vi "UHR-Fleezers Control (host) - 12.1_Jonathan.vi"() -> ()   [LabVIEW 2012] (continued)
  in  "Save Trap Pos. Data":bool=TRUE
  in  "Lower Ch. Cap.":bool
  in  "Top 3 Harvard Syringe Pump Serial Port":refnum<visa-resource-name>="Top3Harvard"
  out "Database link":path
  out "Save Data Period (s)":dbl=0.00375 caption="Period (s)" format="%#_6p"
  out "Save Data Rate (Hz)":dbl=266.6666666666667 caption="Rate (Hz)" format="%#_6p"
  in  "Save ave N":dbl=250.0 caption="Averaging Factor"
  in  "Save N Sets":bool
  in  "N sets to save":u32=200 caption="N Sets"
  out "Total Time (s) 2":dbl=60.0
  # "After"
  # "During"
  # "Trap On?"
  # "BD Flow ON?"
  # "Samp Flow ON?"
  # "Trap Trig. Fl.?"
  # "Zero It"
  # "Floor it\n(e.g., hp unwinding)"
  # "1"
  # "2"
  # "Fl. Down"
  # "Fl. Up"
  # "Bead sep"
  # "Trap Display:"
  # "APD Display:"
  # "DAQ"
  # "Trap Manipulation"
  # "Data Saving"
  # "Bead Calibration"
  # "Bottom Pump (#1)"
  # "Central Sample Channels"
  # "Top Pump (#3)"
  # "Rate param is ul/h\nVolume param is ul"
  # "Chemyx Pump 2"
  # "Units: \n1 = ml/m\n2 = ml/h\n3 = ul/m\n4 = ul/h"
  # "X"
  # "Y"
  # "Oscillate Set 1 freq. (debugging)"
  # "BD 1"
  # "BD 2"
  # "AOD Raster Scan"
  # "Approx. trap separations"
  # "X"
  # "Y"
  # "FPGA\nreading"
  # "DMA\ntransfer"
  # "APD Gates"
  # "APD 2"
  # "APD 1"
  # "X"
  # "2D"
  # "Y"
  # "1D"
  # "Green Laser Interlacing"
  # "Green FB Measurement"
  # "Digital Gate"
  # "Current Analog Control"
  # "Total AI Rates (NOT rates/trap)"
  # "(Samples/trap x Trap Sets)"
  # "(Samples/channel x\n8 if averaging (8 channels)\n4 if no averaging)"
  # "Trap 1"
  # "Trap 2"
  # "Flour./Trap 3"
  # "External Video Window"
  # "MCL Position Debugging"
  # "Temporary Control Storage\n(these used to be somewhere else, still want to keep them)"
  # "Y"
  # "X"
  # "Trap Position Difference Limits"
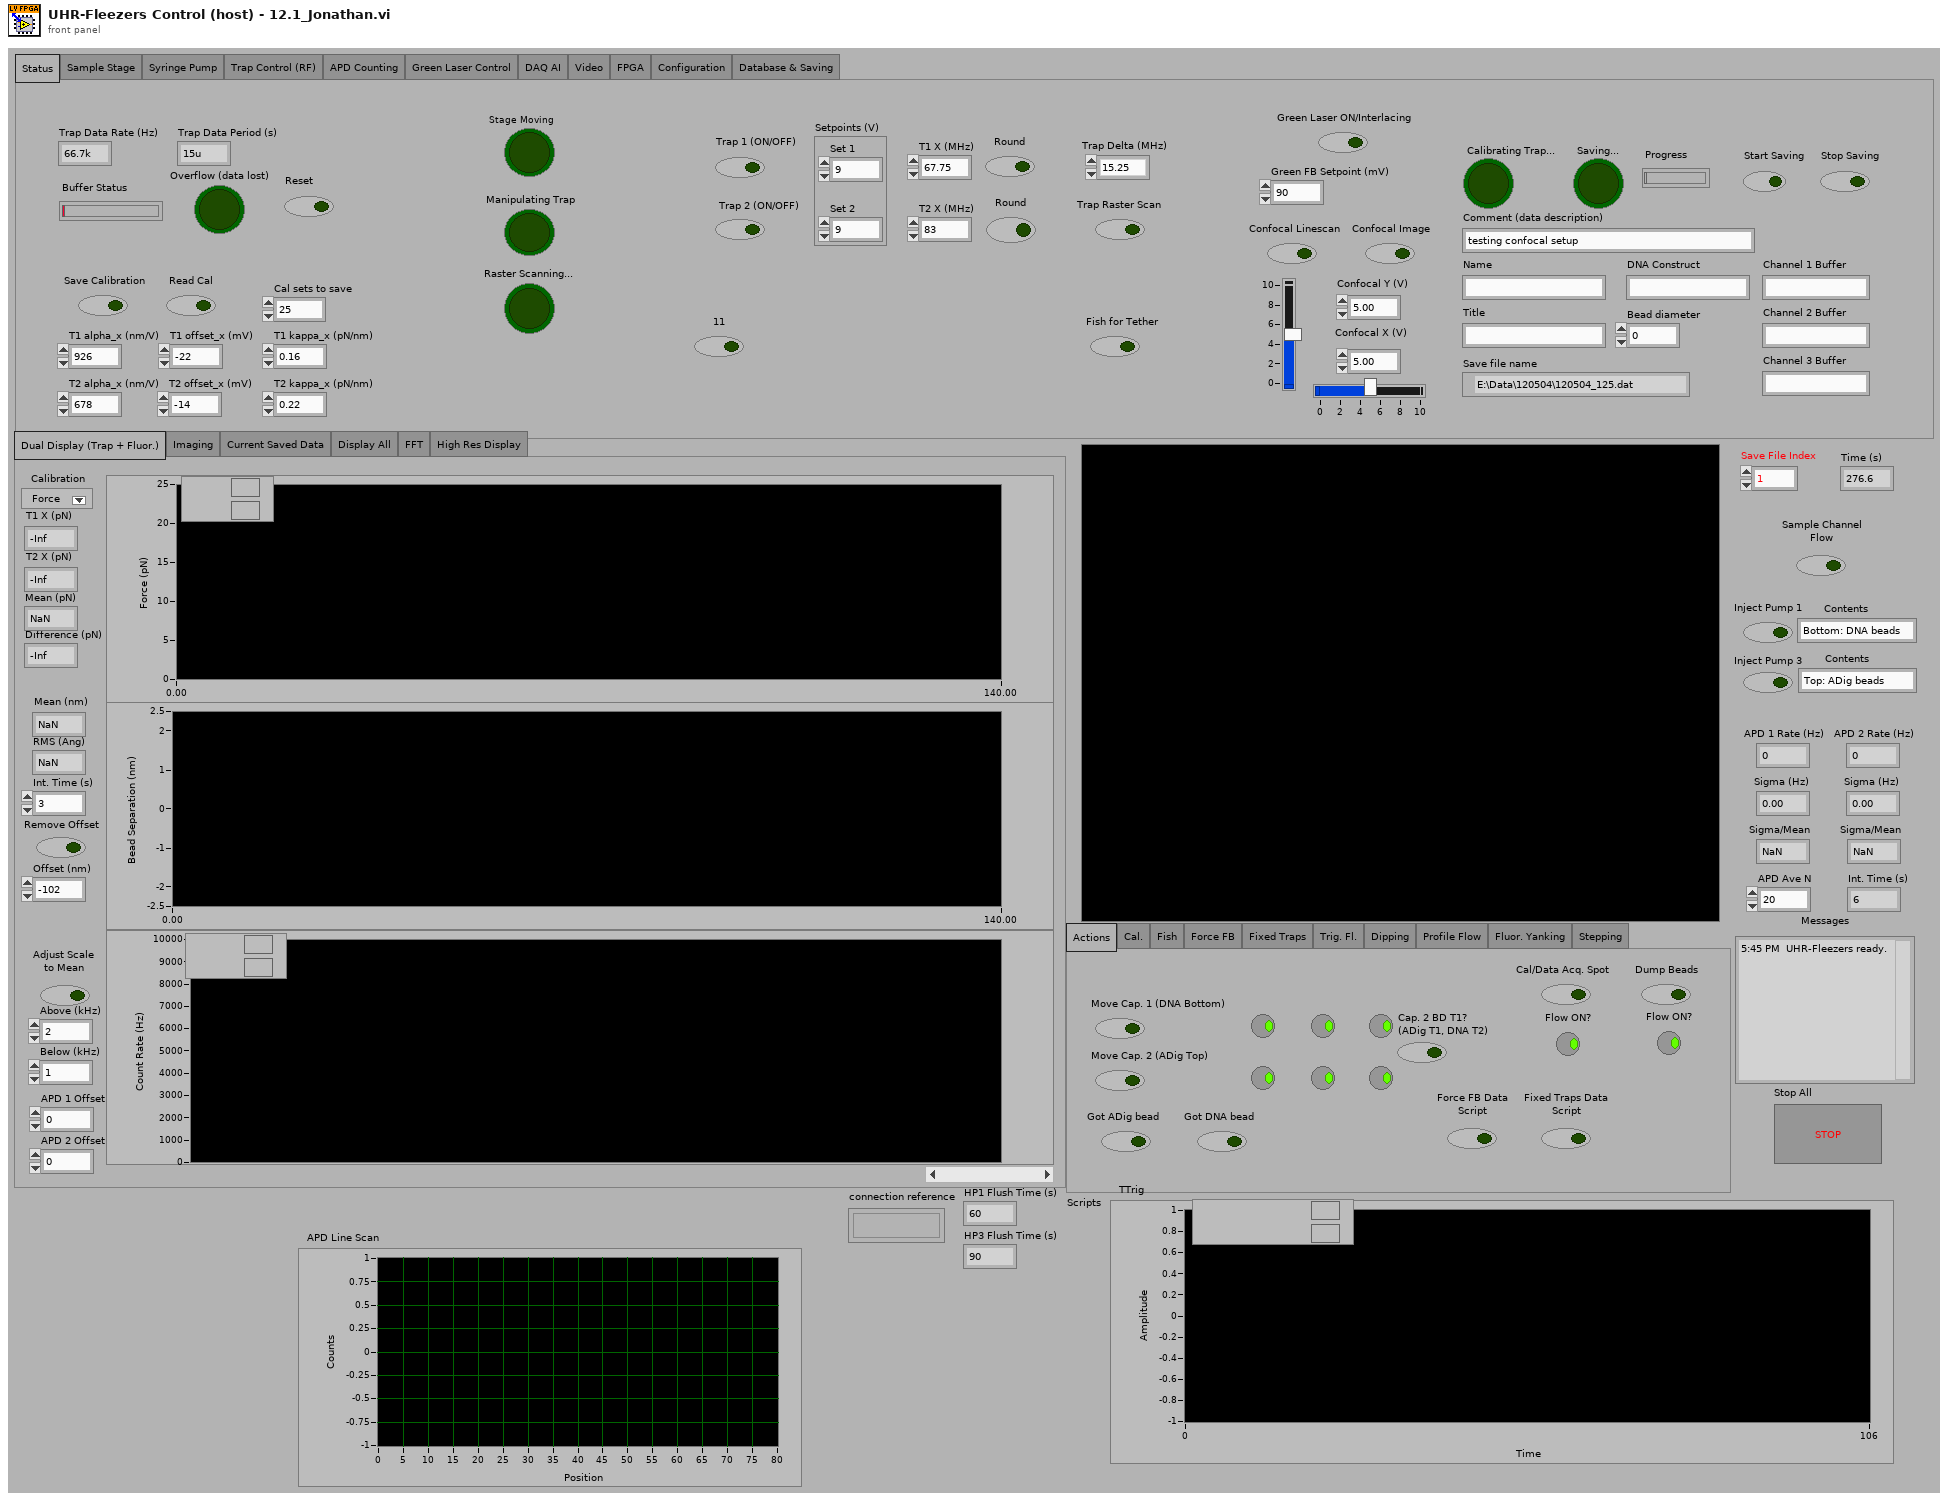
[diagram p1: front panel]
types:
  T1 = typedef "NI_Database_API.lvlib/Conn ObjectReference.ctl" = refnum<k1>
  T2 = enum32{"Actions", "Cal.", "Fish", "Force FB", "Fixed Traps", "Trig. Fl.", "Dipping", "Profile Flow", "Fluor. Yanking", "Stepping"}
  T3 = typedef "IMAQ Image.ctl" = refnum<image>
  T4 = enum32{"Dual Display (Trap + Fluor.)", "Imaging", "Current Saved Data", "Display All", "FFT", "High Res Display"}
  T5 = enum32{"Status", "Sample Stage", "Syringe Pump", "Trap Control (RF)", "APD Counting", "Green Laser Control", "DAQ AI", "Video", "FPGA", "Configuration", "Database & Saving"}
  T6 = cluster{"Pump 1":cluster{"Diameter (mm)":dbl, "Units":dbl, "Volume":dbl, "Rate":dbl}, "Pump 2":cluster{"Diameter (mm)":dbl, "Units":dbl, "Volume":dbl, "Rate":dbl}, "Pump 3":cluster{"Diameter (mm)":dbl, "Units":dbl, "Volume":dbl, "Rate":dbl}}
  T7 = enum32{"IR Laser Interlacing (Direct RF Board Control Method)", "AOD Raster Scan", "Feedback on Trap Intensity", "Feedback on Trap Position"}
  T8 = typedef "LVPoint32TypeDef.ctl" = cluster{"Horizontal":i32, "Vertical":i32}
  T9 = cluster{"Scan Range AOD (nm) 2":dbl, "Step Size AOD (nm) 2":dbl, "Scan Speed AOD (nm/s) 2":dbl, "Number of scans (AOD) 2":u16, "Label":string}[]
  T10 = cluster{"Set 1":cluster{"proportional gain (Kc)":i16, "integral gain (Kc*Ts/Ti)":i16, "derivative gain (Kc*Td/Ts)":i16}, "Set 2":cluster{"proportional gain (Kc)":i16, "integral gain (Kc*Ts/Ti)":i16, "derivative gain (Kc*Td/Ts)":i16}}
  T11 = cluster{"Trap 1":fxp<+/-,16,1>, "Trap 2":fxp<+/-,16,1>}
  T12 = cluster{"proportional gain (Kc)":fxp<+/-,16,8>, "integral gain (Kc*Ts/Ti)":fxp<+/-,16,8>, "derivative gain (Kc*Td/Ts)":fxp<+/-,16,8>}
  T13 = cluster{"output high":fxp<+/-,16,1>, "output low":fxp<+/-,16,1>}
  T14 = cluster{"Set 1":fxp<+/-,16,1>, "Set 2":fxp<+/-,16,1>}
  T15 = cluster{"proportional gain (Kc)":i16, "integral gain (Kc*Ts/Ti)":i16, "derivative gain (Kc*Td/Ts)":i16}
  T16 = cluster{"Set 1":bool, "Set 2":bool, "Set 3":bool}
  T17 = typedef "LVMinMaxIncTypeDef.ctl" = cluster{"Minimum":dbl, "Maximum":dbl, "Increment":dbl}
  T18 = typedef "Image Type" = u32
  T19 = typedef "nirio_resource_hc.ctl" = tag
  T20 = typedef "openfpgaref.8.6.ctl" = refnum<k20>
  T21 = cluster{"New Image":T3, "New Image":T3, "New Image":T3, "New Image":T3}
  T22 = typedef "XDNodeRunTimeDep.lvlib/timing_clust.ctl" = cluster{"Expected End [f-1]":u64, "Actual End [f-1]":u64, "Finished Late? [f-1]":bool, "Expected End [i-1]":u64, "Actual End [i-1]":u64, "Finished Late? [i-1]":bool, "Expected Start [i]":u64, "Actual Start [i]":u64, "Expected Start [f]":u64, "Actual Start [f]":u64, "Source Name":string, "Structure Name":string, "Period":i64, "Deadline":i64, "Offset":i64, "Start":i64, "Priority":i32, "Timeout":i32, "Mode":T23, "Wakeup Reason":T24, "Error":errorcluster, "Source Type":string, "Secondary Source Type":string, "Global End Time":u64, "Global Start Time":u64, "Frame Duration":u64, "Iteration Duration":u64, "Assigned CPU":i32, "I/O Scan Engine Mode":u32}
  T23 = typedef "XDNodeRunTimeDep.lvlib/nitl_modes.ctl" = enum32{"No Change", "Process missed periods, maintain original phase", "Discard missed periods, maintain original phase", "Process missed periods, ignore original phase", "Discard missed periods, ignore original phase"}
  T24 = typedef "XDNodeRunTimeDep.lvlib/wakeup.ctl" = enum32{"Normal", "Aborted", "Asynchronous wakeup", "Timing source error", "Timed loop error", "Timeout"}
  T25 = cluster{"Left":i32, "Top":i32, "Width":u32, "Height":u32}
  T26 = cluster{cluster{"Left":i32, "Top":i32, "Width":u32, "Height":u32}}[]
  T27 = enum32{"Status", "Sample Stage", "Syringe Pump", "Trap Control (RF)", "APD Counting", "Green Laser Control", "DAQ AI", "Video", "FPGA", "Configuration"}
  T28 = enum32{"setting", "request", "request control", "info", "statistics", "system settings", "I/O sub system", "HRT control", "camera descriptions", "device specific data", "event sub system settings", "event sub system results", "image memory manager"}
  T29 = typedef "AviRefnum.ctl" = refnum<k1>
  T30 = typedef "imagedata.ctl" = cluster{"image type":i32, "image depth":i32, "image":u8[], "mask":u8[], "colors":u32[], "Rectangle":cluster{"left":i16, "top":i16, "right":i16, "bottom":i16}}
  T31 = enum32{"Normal Display", "Dual Display (APD)", "FFT", "High Res Display"}
  T32 = cluster{"Origin Pixel":cluster{"X":sgl, "Y":sgl}, "Angle Relative to Horizontal (deg)":sgl, "Axis Reference":u32}
  T33 = typedef "Simple Grid Descriptor" = cluster{"X Step":sgl, "Y Step":sgl, "Unit":T34}
  T34 = typedef "Image Unit" = enum32{"Undefined", "Angström", "Micrometer", "Millimeter", "Centimeter", "Meter", "Kilometer", "Microinch", "Inch", "Feet", "Nautical miles", "Standard miles", "Steps"}
  T35 = cluster{"averaging mode":u16, "weighting mode":u16, "number of averages":u32}
  T36 = cluster{"dB On (F)":bool, "unwrap phase (F)":bool, "convert to degree (F)":bool}
  T37 = enum16{"open", "replace", "create", "open or create", "replace or create", "replace or create with confirmation"}
  T38 = enum16{"big-endian, network order", "native, host order", "little-endian"}
  T39 = cluster{string, string, string, string, string, string, string, string}
  T40 = cluster{string, string, string, string, string, string, string, string, string, string, string, string}
  T41 = cluster{string, string, string, string, string, string, string, string, string, string, string, string, string}
  T42 = cluster{string, string, string, string, string, string, string, string, string, string, string, string, string, string}
  T43 = cluster{"BD 1 Frequency 1 (MHz)":dbl, "BD 1 Frequency 2 (MHz)":dbl}
  T44 = cluster{"f0":dbl, "df":dbl, "magnitude":dbl[]}[][]
  T45 = cluster{"Green FB Ch 0":i16, "Green FB Ch 1":i16, "Green FB Ch 2":i16}
  T46 = cluster{"Green FB Ch 0":dbl, "Green FB Ch 1":dbl, "Green FB Ch 2":dbl}
  T47 = cluster{"Comment (data description)":string, "Channel 1 Buffer":string, "Channel 2 Buffer":string, "Channel 3 Buffer":string, "Title":string, "DNA Construct":string, "Bead diameter":dbl, "Name":string}
  T48 = cluster{"Scan Range AOD (nm) 2":dbl, "Step Size AOD (nm) 2":dbl, "Scan Speed AOD (nm/s) 2":dbl, "Number of scans (AOD) 2":u16, "Label":string}
  T49 = cluster{"[0]":dbl, "[1]":dbl, "[2]":dbl, "[3]":dbl, "[4]":dbl, "[5]":dbl}
  T50 = cluster{"Diameter (mm)":dbl, "Units":dbl, "Volume":dbl, "Rate":dbl}
diagram:
  w14 = u16 20 items=["1.0"=10, "1.5"=15, "2.0"=20] ("stop bits (10: 1 bit)")
  w17 = u16 20 items=["1.0"=10, "1.5"=15, "2.0"=20] ("stop bits (10: 1 bit)")
  w74 = u16 20 items=["1.0"=10, "1.5"=15, "2.0"=20] ("stop bits (10: 1 bit)")
  w81 = T18 2 items=["Grayscale (U8)", "Grayscale (I16)", "Grayscale (SGL)", "Complex (CSG)", "RGB (U32)", "HSL (U32)", "RGB (U64)", "Grayscale (U16)"] ("Image Type")
  w143 = cluster{"output high":i16, "output low":i16} {"output high"=3000, "output low"=0} ("FB output range 1")
  w214 = 10.0 ("y")
  w213 = 32767.0 ("y")
  w229 = 6.0  # clock mult.
  w230 = 49152000.0  # TCXO frequ.
  # "Bottom 1 Harvard"
  # "Top 3 Harvard"
  # "Center Harvard"
  # "Bottom 1 Harvard"
  # "Top 3 Harvard"
  # "Center Harvard"
  n1 = Build Array("DIO count 1 (ticks)", "DIO count 2 (ticks)", "DIO count 3 (ticks)") -> (w131:u32[])
  n2 = local read "AO1"() -> (w208:dbl)
  n3 = local read "AO2"() -> (w207:dbl)
  n4 = local read "Scan Increment (MHz)"() -> (w225:dbl)
  n5 = local read "Continuous MCL Scanning"() -> (w195:bool)
  n6 = local read "Fast Scan Dir"() -> (w194:bool)
  n7 = local read "Number of scans (MCL)"() -> (w196:u64)
  n8 = property on="AI Count (ticks)" class="DigNum (strict)"("Val(Sgnl)"="AI Count (ticks)") -> ()  [unwired: 2 in, 2 out]
  n9 = Multiply(x=w208, y=w213) -> (x*y=w210:dbl)
  n10 = Multiply(x=w207, y=w213) -> (x*y=w212:dbl)
  n11 = Divide(x=w210, y=w214) -> (x/y=w209:dbl)
  n12 = Divide(x=w212, y=w214) -> (x/y=w211:dbl)
  n13 = To Word Integer(number=w209) -> (16bit integer=w206:i16)
  n14 = To Word Integer(number=w211) -> (16bit integer=w205:i16)
  n15 = Not(x=w194) -> (.not. x?=w189:bool)
  n16 = local read "Cycles/step (MCL)"() -> (w197:u64)
  n17 = Multiply(x=w225, y=1000.0) -> (x*y=w232:dbl)
  n18 = local read "Scan steps (MCL)"() -> (w198:u64)
  n19 = local write "Trap Pos FIFO Timeout"(u16 0 ("Trap Pos FIFO Timeout")) -> ()
  n20 = local read "Desired Scan Incr (V)"() -> (w200:dbl)
  n21 = Scale By Power Of 2(n=48, x=w232) -> (x*2^n=w233:dbl)
  n22 = Multiply(x=w230, y=w229) -> (x*y=w228:dbl)
  n23 = Divide(x=w233, y=w228) -> (x/y=w227:dbl)
  n24 = local read "Setpoints (V)"() -> (w246:cluster{"Set 1":dbl, "Set 2":dbl})
  n25 = To Quad Integer(1:w227) -> (0:w224:i64)
  n26 = Divide(x=40000000.0, y="AI Count (ticks)") -> (x/y=w185:dbl)
  n27 = Multiply(x=w200, y=32767.0) -> (x*y=w202:dbl)
  n28 = local read "Number Interlace Sets"() -> (w124:u8)
  n29 = Split 1D Array(array=w131, index=w124) -> (first subarray=w133:u32[])  [unwired: 1 out]
  n30 = Add Array Elements(numeric array=w133) -> (sum=w132:u32)
  n31 = local read "# Samples/channel"() -> (w217:u32)
  n32 = local read "Number of F/B Scans (AOD)"() -> (w218:u16)
  n33 = local read "Not-Interlacing Set"() -> (w123:enum32{"Set 1", "Set 2", "Set 3"})
  n34 = To Unsigned Byte Integer(number=w123) -> (unsigned 8bit integer=w129:u8)
  n35 = Index Array(array=w131, index=w129) -> (element=w130:u32)
  n36 = local read "Feedback On/Off"() -> (w249:cluster{"Set 1":bool, "Set 2":bool})
  n37 = local read "PID Gains"() -> (w241:T10)
  n38 = local read "Scan steps (AOD)"() -> (w223:u64)
  n39 = local read "All FB On/Off"() -> (w250:bool)
  n40 = local read "Cycles/step (AOD)"() -> (w222:u64)
  n41 = local write "AI rate (Hz)"(w185) -> ()
  n42 = Divide(x=w202, y=10.0) -> (x/y=w201:dbl)
  n43 = Multiply(x=w223, y=w222) -> (x*y=w221:u64)
  n44 = Multiply(x=3276.7, y=w246) -> (x*y=w245:cluster{"Set 1":dbl, "Set 2":dbl})
  n45 = xnode "FPGA Open VI Reference"("resource name"=T19 "750kHzDAQ") -> ("FPGA VI Reference Out"=w238:T20, "error out"=w237:errorcluster)  [unwired: 1 in]
  n46 = To Word Integer(number=w201) -> (16bit integer=w199:i16)
  n47 = Multiply(x=w221, y=u64 2) -> (x*y=w219:u64)
  n48 = local read "Sets to FIFO (Traps)"() -> (w253:T16)
  n49 = Divide(x=w185, y="FPGA Ave.") -> (x/y=w186:dbl)
  n50 = To Word Integer(number=w245) -> (16bit integer=w244:cluster{"Set 1":i16, "Set 2":i16})
  n51 = Unbundle By Name(w241) -> ("Set 1"=w240:T15, "Set 2"=w239:T15)
  n52 = Multiply(x=w219, y=w218) -> (x*y=w216:u64)
  n53 = local write "Ave. Rate (Hz)"(w186) -> ()
  n54 = Divide(x=w216, y=w217) -> (x/y=w215:dbl)
  n55 = Unbundle By Name(w244) -> ("Set 1"=w243:i16, "Set 2"=w242:i16)
  n56 = local read "2D or 1D Scan"() -> (w144:bool)
  n57 = local write "Data points/scans"(w216) -> ()
  n58 = local read "Scan BD"() -> (w234:bool)
  n59 = And(x=w249, y=w250) -> (x .and. y?=w248:cluster{"Set 1":bool, "Set 2":bool})
  n60 = local write "Data points/scan (f/b)"(w219) -> ()
  n61 = Reciprocal(x=w186) -> (1/x=w187:dbl)
  n62 = local read "N Acq Sets (Traps + Fl.)"() -> (w178:i16)
  n63 = local write "N sets should be saved"(w215) -> ()
  n64 = xnode "Invoke Method"("FPGA VI Reference In"=w238, "error in"=w237) -> ("FPGA VI Reference Out"=w142:T20, "error out"=w152:errorcluster)
  n65 = Unbundle By Name(w248) -> ("Set 1"=w252:bool, "Set 2"=w251:bool)
  n66 = local read "Interlace"() -> (w125:bool)
  n67 = Select(t=w132, s=w125, f=w130) -> (s? t:f=w122:u32)
  n68 = local write "Update Count (MCL)"(w122) -> ()
  n69 = local write "Total Counts (ticks)"(w122) -> ()
  n70 = local write "Ave. Period (s)"(w187) -> ()
  n71 = property on="2D or 1D Scan" class="Bool (strict)"("Val(Sgnl)"=w144) -> ()  [unwired: 2 in, 2 out]
  n72 = local read "GI Frequency, OFF count"() -> (w46:u32)
  n73 = local read "GI Frequency, ON count"() -> (w37:u32)
  n74 = local read "APD Gate OFF Count"() -> (w43:u32)
  n75 = local read "APD Gate ON Count"() -> (w39:u32)
  n76 = xnode "Read/Write Control"("FPGA VI Reference In"=w141, "error in"=w152, "ai count"="AI Count (ticks)", "Interlace ON/OFF"=w125, "Number Interlace Cycles"=w124, "AI1 Sets to FIFO"=w253, "FB On/Off Set 1"=w252, "FB On/Off Set 2"=w251, "Interlace Off Parameters"=w123, "FB Setpoint Set 1"=w243, "FB Setpoint Set 2"=w242, "FB Gains Set 1"=w240, "FB Gains Set 2"=w239, "FB output range 1"=w143, "FB output range 2"=w143, "Cycles per step"=w222, "Scan BD"=w234, "Number of scans"=w218, "Scan steps"=w223, "Scan freq.  increment"=w224, "AO1"=w206, "AO2"=w205, "Scan freq.  increment (MCL)"=w199, "Scan steps (MCL)"=w198, "Cycles per step (MCL)"=w197, "Number of scans (MCL)"=w196, "MCL count"=w122, "Cont. Scan (MCL)"=w195, "MCL Scan Axis"=w189, "1D or 2D Scan?"=w144, "N of AI1 Int Acq Sets"=w178, "Freq or Amp switch first"="Freq or Amp switch first", "Freq switch delay"="Freq switch delay", "Amp switch delay"="Amp switch delay", "Swap F1 and F2"="Swap F1 and F2", "APD to FIFO"=FALSE, "DIO count 1 (ticks)"="DIO count 1 (ticks)", "DIO count 2 (ticks)"="DIO count 2 (ticks)", "DIO count 3 (ticks)"="DIO count 3 (ticks)") -> ("FPGA VI Reference Out"=w50:T20, "error out"=w48:errorcluster)  [unwired: 1 in]
  n77 = local read "On one out of X cycles"() -> (w45:u32)
  n78 = local read "APD Integration Time (s)"() -> (w29:dbl)
  n79 = local read "DMA Update Period (s)"() -> (w28:dbl)
  n80 = Add(x=w39, y=w43) -> (x+y=w41:u32)
  n81 = Add(x=w37, y=w46) -> (x+y=w44:u32)
  n82 = local read "Green Laser ON/Interlacing"() -> (w120:bool)
  n83 = local read "Green laser mode"() -> (w121:enum32{"Laser ON", "Laser OFF", "Interlace"})
  n84 = Multiply(x=w41, y=w45) -> (x*y=w42:u32)
  n85 = Multiply(x=w45, y=w44) -> (x*y=w36:u32)
  n86 = Reciprocal(x=w29) -> (1/x=w26:dbl)
  n87 = Multiply(x=w29, y=40000000.0) -> (x*y=w25:dbl)
  n88 = Divide(x=w28, y=w29) -> (x/y=w31:dbl)
  n89 = Multiply(x="Current When FB OFF (%)", y=655.35) -> (x*y=w108:dbl)
  n90 = local read "Invert APD Gate"() -> (w35:bool)
  n91 = Multiply(x="Green FB Setpoint (mV)", y=3.2767) -> (x*y=w105:dbl)
  n92 = local read "APD Gate"() -> (w34:enum32{"ON", "OFF", "Interlace"})
  n93 = Subtract(x=w42, y=w39) -> (x-y=w40:u32)
  n94 = local write "Green FB Count"(w36) -> ()
  n95 = local write "APD Acq Rate (Hz)"(w26) -> ()
  n96 = To Unsigned Long Integer(number=w25) -> (unsigned 32bit integer=w23:u32)
  n97 = Multiply(x=2.0, y=w31) -> (x*y=w30:dbl)
  n98 = local read "Invert GI"() -> (w117:bool)
  n99 = To Unsigned Word Integer(number=w108) -> (unsigned 16bit integer=w106:u16)
  n100 = Subtract(x=w36, y=w37) -> (x-y=w38:u32)
  n101 = local write "APD Samples/FIFO Acq."(w31) -> ()
  n102 = To Word Integer(number=w105) -> (16bit integer=w103:i16)
  n103 = local write "APD Elements/DMA read"(w30) -> ()
  n104 = case shown="False" w120 {
    tunnel: w121 -> [_ w279]
    tunnel: [enum32{"Laser ON", "Laser OFF", "Interlace"}."Laser OFF" ("Green laser mode") w279] -> w116
    frame False {
    }
    frame True {
    }
  }
  n105 = local write "APD Int. Count"(w23) -> ()
  n106 = local read "Trap Pos. AI1 X Pre-scale"() -> (w60:u16)
  n107 = local read "Trap Pos FB Monitor\nT1 or T2"() -> (w67:bool)
  n108 = local read "Trap Pos FB Int Count"() -> (w54:u16)
  n109 = local read "APD 1 AO Mult."() -> (w33:i16)
  n110 = local read "Trap Pos FB Negate Action"() -> (w66:bool)
  n111 = local read "APD 2 AO Mult."() -> (w32:i16)
  n112 = local read "Trap Pos. FB Offset Factor"() -> (w65:i64)
  n113 = local read "Trap Pos. FB Mult Factor"() -> (w64:i64)
  n114 = local read "Differential FB?"() -> (w20:bool)
  n115 = local read "Neg. TTrig FPGA"() -> (w22:bool)
  n116 = local read "Trap Pos. FB Gains"() -> (w62:T12)
  n117 = local read "Trap Pos. FB Range"() -> (w63:T13)
  n118 = xnode "Read/Write Control"("FPGA VI Reference In"=w50, "error in"=w48, "Invert APD Gate"=w35, "APD Gate ON Count"=w39, "APD Gate OFF Count"=w40, "APD Acq Rate Count"=w23, "APD Gate Operating Mode"=w34, "APD 1 AO scale factor"=w33, "APD 2 AO scale factor"=w32, "Green interlace ON count"=w37, "Green interlace OFF count"=w38, "Green interlace ON count 2"=w37, "Green interlace OFF count 2"=w38, "Green FB Count"=w36) -> ("FPGA VI Reference Out"=w49:T20, "error out"=w47:errorcluster)
  n119 = xnode "Read/Write Control"("FPGA VI Reference In"=w49, "error in"=w47, "Invert GI 2"=w117, "Operating Mode 2"=w116, "Green FB Gains"="Green FB Gains", "Green FB Setpoint"=w103, "Green FB On/Off"="Green FB On/Off", "Current Out"=w106, "Green int current ON count adj"="Green int current ON count adj", "Operating Mode"=w116, "Invert GI"=w117, "Trap Pos FB Monitor T1 or T2"=w67, "Trap Pos FB Negate Action"=w66, "Trap Pos. FB Offset Factor"=w65, "Trap Pos. FB Mult Factor"=w64, "Trap Pos. FB Range"=w63, "Trap Pos. FB Gains"=w62, "Force feedback"=FALSE, "AI1 X Scale"=w60, "Trap Pos to FIFO"=TRUE, "Trap Pos FB Int Count"=w54, "TTrig Negate Pos"=w22, "FB Trig Integrate"="FB Trig Integrate", "Diff FB Measurement?"=w20, "Negate Diff?"="Negate Diff?") -> ("FPGA VI Reference Out"=w118:T20, "error out"=w119:errorcluster)
  n120 = xnode "Invoke Method"("FPGA VI Reference In"=w118, "error in"=w119, "Requested Depth"="Trap AI FIFO Depth") -> ("FPGA VI Reference Out"=w70:T20, "error out"=w69:errorcluster)  [unwired: 1 out]
  n121 = xnode "Invoke Method"("FPGA VI Reference In"=w70, "error in"=w69, "Requested Depth"="Trap Position FIFO Depth") -> ("FPGA VI Reference Out"=w56:T20, "error out"=w55:errorcluster)  [unwired: 1 out]
  n122 = flat-sequence {
    tunnel: w142 -> [w284]
    tunnel: [w284] -> w141
    tunnel: [w283] -> w140
    tunnel: [w282] -> w139
    tunnel: [w280] -> w137
    tunnel: [w281] -> w138
    frame #0 {
      w281 = T17 {"Minimum"=0.0, "Maximum"=40.0, "Increment"=1.0} ("Min Max Inc")
      w280 = T17 {"Minimum"=0.0, "Maximum"=50.0, "Increment"=1.0} ("Data Entry Limits")
      w283 = T17 {"Minimum"=60.0, "Maximum"=90.0, "Increment"=1.0} ("Min Max Inc")
      w282 = T17 {"Minimum"=0.0, "Maximum"=50.0, "Increment"=1.0} ("Data Entry Limits")
      n123 = property on="BD 2 Frequency 1 (MHz)" class="DigNum (strict)"("Data Range"=w281) -> ()  [unwired: 2 in, 2 out]
      n124 = property on="BD 2 Frequency 3 (MHz)" class="DigNum (strict)"("Data Range"=w281) -> ()  [unwired: 2 in, 2 out]
      n125 = property on="BD 2 Frequency 2 (MHz)" class="DigNum (strict)"("Data Range"=w281) -> ()  [unwired: 2 in, 2 out]
      n126 = property on="BD 1 Frequency 1 (MHz)" class="DigNum (strict)"("Data Range"=w283) -> ()  [unwired: 2 in, 2 out]
      n127 = property on="BD 1 Frequency 2 (MHz)" class="DigNum (strict)"("Data Range"=w283) -> ()  [unwired: 2 in, 2 out]
      n128 = property on="BD 1 Frequency 3 (MHz)" class="DigNum (strict)"("Data Range"=w283) -> ()  [unwired: 2 in, 2 out]
      n129 = property on="BD 2 Amplitude 1 (%)" class="DigNum (strict)"("Data Range"=w280) -> ()  [unwired: 2 in, 2 out]
      n130 = property on="BD 2 Amplitude 2 (%)" class="DigNum (strict)"("Data Range"=w280) -> ()  [unwired: 2 in, 2 out]
      n131 = property on="BD 2 Amplitude 3 (%)" class="DigNum (strict)"("Data Range"=w280) -> ()  [unwired: 2 in, 2 out]
      n132 = property on="BD 1 Amplitude 3 (%)" class="DigNum (strict)"("Data Range"=w282) -> ()  [unwired: 2 in, 2 out]
      n133 = property on="BD 1 Amplitude 2 (%)" class="DigNum (strict)"("Data Range"=w282) -> ()  [unwired: 2 in, 2 out]
      n134 = property on="BD 1 Amplitude 1 (%)" class="DigNum (strict)"("Data Range"=w282) -> ()  [unwired: 2 in, 2 out]
      "X RF Frequency Limits (MHz)" <- w283
      "X RF Amplitude Limits (%)" <- w282
      "Y RF Amplitude Limits (%)" <- w280
      "Y RF Frequency Limits (MHz)" <- w281
    }
  }
  n135 = xnode "Invoke Method"("FPGA VI Reference In"=w56, "error in"=w55) -> ("FPGA VI Reference Out"=w151:T20, "error out"=w150:errorcluster)  [unwired: 1 in]
  n136 = flat-sequence "Initial FPGA Loop Relative Phase Adjustment" {
    tunnel: "Initial Phase Adjustment (AI1)" -> [w295]
    tunnel: "Initial Phase Adjustment (GI)" -> [w294]
    tunnel: w151 -> [w293]
    tunnel: w150 -> [w292]
    tunnel: "Initial Phase Adj. (MCL)" -> [w291]
    tunnel: [w296] -> w160
    tunnel: [w290] -> w156
    tunnel: "Initial Phase Adjustment (APD Acq)" -> [w289]
    tunnel: "Initial Phase Adjustment (APD 1 Gate)" -> [w288]
    tunnel: "Initial Phase Adjustment (Green FB)" -> [w287]
    tunnel: "Initial Phase Adjustment (GI) 2" -> [w286]
    tunnel: "Initial Phase Adjustment (APD 2 Gate)" -> [w285]
    tunnel: w160 -> [w298]
    tunnel: [w299] -> w157
    tunnel: w156 -> [w299]
    tunnel: [w298] -> w155
    tunnel: w157 -> [w302]
    tunnel: w155 -> [w301]
    tunnel: [w304] -> w154
    tunnel: [w303] -> w153
    tunnel: [w306] -> w158
    tunnel: [w307] -> w159
    tunnel: w154 -> [w307]
    tunnel: w153 -> [w306]
    frame #0 {
      n137 = xnode "Read/Write Control"("FPGA VI Reference In"=w293, "error in"=w292, "Phase count adjustment"=w295, "Phase count adjustment (GI)"=w294, "Phase count adjustment (MCL)"=w291, "Phase Count Adjustment (APD Acq)"=w289, "Phase count adjustment (APD 1 Gate)"=w288, "Phase count adjustment (APD 2 Gate)"=w285, "Phase count adjustment (Green FB)"=w287, "Phase count adjustment (GI) 2"=w286) -> ("FPGA VI Reference Out"=w290:T20, "error out"=w296:errorcluster)
    }
    frame #1 {
      n138 = Wait (ms)(milliseconds to wait=u32 100) -> ()  [unwired: 1 out]
    }
    frame #2 {
      w300 = TRUE
      n139 = xnode "Read/Write Control"("FPGA VI Reference In"=w302, "error in"=w301, "+ phase"=w300, "+ phase (GI)"=w300, "+ phase (MCL)"=w300, "+ phase (APD Acq)"=w300, "+ phase (APD 1 Gate)"=w300, "+ phase (APD 2 Gate)"=w300, "+ phase (Green FB)"=w300, "+ phase (GI) 2"=w300) -> ("FPGA VI Reference Out"=w303:T20, "error out"=w304:errorcluster)
    }
    frame #3 {
      n140 = Wait (ms)(milliseconds to wait=u32 100) -> ()  [unwired: 1 out]
    }
  }
  n141 = local read "Phase adj. (Green FB)"() -> (w134:i16)
  n142 = local read "Phase adj. (GI) 2"() -> (w109:i16)
  n143 = local read "Phase adjust (MCL)"() -> (w190:i16)
  n144 = local read "Phase adj. (AI1)"() -> (w192:i16)
  n145 = local read "Phase adj. (GI)"() -> (w191:i16)
  n146 = xnode "Read/Write Control"("FPGA VI Reference In"=w158, "error in"=w159, "Phase count adjustment"=w192, "Phase count adjustment (GI)"=w191, "Phase count adjustment (MCL)"=w190, "Phase Count Adjustment (APD Acq)"="Phase Adj. (APD Acq)", "Phase count adjustment (APD 1 Gate)"="Phase Adj. (APD 1 Gate)", "Phase count adjustment (APD 2 Gate)"="Phase Adj. (APD 2 Gate)", "Phase count adjustment (Green FB)"=w134, "Phase count adjustment (GI) 2"=w109) -> ("FPGA VI Reference Out"=w95:T20, "error out"=w167:errorcluster)
  n147 = call "Initialize RF boards - interlace 3.vi"("error in"=w167, "FPGA VI Reference In"=w95) -> ("error out"=w165:errorcluster, "FPGA VI Reference Out"=w166:T20)
  n148 = call "set RF board frequency - interlace.vi"("Board 2 Frequency Limits"=w138, "Board 1 Frequency Limits"=w140, "error in"=w165, "FPGA VI Reference In"=w166, "Board 2 Frequency 3 (MHz)"="BD 2 Frequency 3 (MHz)", "Board 1 Frequency 3 (MHz)"="BD 1 Frequency 3 (MHz)", "Board 2 Frequency 2 (MHz)"="BD 2 Frequency 2 (MHz)", "Board 2 Frequency 1 (MHz)"="BD 2 Frequency 1 (MHz)", "Board 1 Frequency 2 (MHz)"="BD 1 Frequency 2 (MHz)", "Board 1 Frequency 1  (MHz)"="BD 1 Frequency 1 (MHz)") -> ("error out"=w268:errorcluster, "FPGA VI Reference Out"=w269:T20)
  n149 = call "set RF board amplitude - interlace.vi"("Board 2 Amplitude Limits"=w137, "Board 1 Amplitude Limits"=w139, "error in"=w268, "FPGA VI Reference In"=w269, "Board 2 Amplitude 3 (%)"="BD 2 Amplitude 3 (%)", "Board 1 Amplitude 3 (%)"="BD 1 Amplitude 3 (%)", "Board 2 Amplitude 2 (%)"="BD 2 Amplitude 2 (%)", "Board 2 Amplitude 1 (%)"="BD 2 Amplitude 1 (%)", "Board 1 Amplitude 2 (%)"="BD 1 Amplitude 2 (%)", "Board 1 Amplitude 1 (%)"="BD 1 Amplitude 1 (%)") -> ("error out"=w256:errorcluster, "FPGA VI Reference Out"=w257:T20)
  n150 = flat-sequence {
    tunnel: w257 -> [w317]
    tunnel: w256 -> [w316]
    tunnel: [w315] -> w261
    tunnel: [w314] -> w260
    tunnel: [w321] -> w259
    tunnel: w261 -> [w321]
    tunnel: [w320] -> w258
    tunnel: w260 -> [w320]
    tunnel: w259 -> [w330]
    tunnel: w258 -> [w329]
    tunnel: [w328] -> w2
    tunnel: [w327] -> w1
    tunnel: [w334] -> w57
    tunnel: [w335] -> w8
    tunnel: w2 -> [w335]
    tunnel: w1 -> [w334]
    frame #0 {
      w308 = FALSE ("Retract Pump 3")
      n151 = local read "Trap 1 (ON/OFF)"() -> (w309:bool)
      n152 = xnode "Read/Write Control"("FPGA VI Reference In"=w317, "error in"=w316, "Direct RF Box  Communication"=FALSE) -> ("FPGA VI Reference Out"=w315:T20, "error out"=w314:errorcluster)
      n153 = local write "Saving..."(FALSE ("Saving Data")) -> ()
      n154 = local write "Stop All"(FALSE ("Stop All")) -> ()
      n155 = local write "Retract Pump 1"(w308) -> ()
      n156 = local write "Retract Pump 3"(w308) -> ()
      n157 = local write "Index"(1.0 ("Index")) -> ()
      n158 = property on="Trap 1 ON" class="Bool (strict)"("Value"=w309) -> ()  [unwired: 2 in, 2 out]
      "Manipulating Trap" <- FALSE ("Manipulating Trap")
    }
    frame #1 {
      n159 = local read "Trap 2 (ON/OFF)"() -> (w319:bool)
      n160 = Wait (ms)(milliseconds to wait=u32 10) -> ()  [unwired: 1 out]
      n161 = property on="Trap 2 ON" class="Bool (strict)"("Val(Sgnl)"=w319) -> ()  [unwired: 2 in, 2 out]
    }
    frame #2 {
      n162 = local read "Scan Range (nm)"() -> (w323:dbl)
      n163 = xnode "Read/Write Control"("FPGA VI Reference In"=w330, "error in"=w329, "FPGA Controls  RF Box"=TRUE ("Direct RF Box  Communication")) -> ("FPGA VI Reference Out"=w328:T20, "error out"=w327:errorcluster)
      n164 = call "Update messages.vi"("Message to add"="UHR-Fleezers ready.", "Old message string"="") -> ("New message string"=w326:string)
      n165 = local write "Messages"(w326) -> ()
      n166 = property on="Scan Range (nm)" class="DigNum (strict)"("Val(Sgnl)"=w323) -> ()  [unwired: 2 in, 2 out]
    }
    frame #3 {
      w332 = path "C:/Home/wheeler/Comstock-LabView-Link.udl" ("connection information")
      n167 = local write "Database link"(w332) -> ()
      n168 = call-poly <vilib>:"DB Tools Open Connection.vi"("connection information"=w332) -> ("connection reference"=w333:T1)  [unwired: 7 in, 1 out]
      "connection reference" <- w333
      n169 = local write "connection reference"(w333) -> ()
    }
  }
  n170 = Subtract(x="BD 1 Frequency 1 (MHz)", y="BD 1 Frequency 2 (MHz)") -> (x-y=w177:dbl)
  n171 = Subtract(x="BD 2 Frequency 1 (MHz)", y="BD 2 Frequency 2 (MHz)") -> (x-y=w176:dbl)
  n172 = Square(x=w176) -> (x^2=w174:dbl)
  n173 = Square(x=w177) -> (x^2=w175:dbl)
  n174 = Add(x=w175, y=w174) -> (x+y=w173:dbl)
  n175 = Square Root(x=w173) -> (sqrt(x)=w172:dbl)
  n176 = local write "Trap Delta (MHz)"(w172) -> ()
  n177 = call "IMAQ Create"("Image Name"="APD 1 Image", "Image Type"=w81) -> ("New Image"=w80:T3)  [unwired: 3 in, 1 out]
  n178 = call "IMAQ Create"("Image Name"="APD 2 Image", "Image Type"=w81) -> ("New Image"=w79:T3)  [unwired: 3 in, 1 out]
  n179 = call "IMAQ Create"("Image Name"="Det. X Image", "Image Type"=w81) -> ("New Image"=w78:T3)  [unwired: 3 in, 1 out]
  n180 = call "IMAQ Create"("Image Name"="Det. Y Image", "Image Type"=w81) -> ("New Image"=w77:T3)  [unwired: 3 in, 1 out]
  n181 = Bundle("New Image"=w80, "New Image"=w79, "New Image"=w78, "New Image"=w77) -> (w76:T21)  [unwired: 1 in]
  n182 = call-poly "VISA Configure Serial Port"("VISA resource name"="Bottom  1 Harvard Syringe Pump Serial Port", "baud rate (9600)"=u32 115200, "stop bits (10: 1 bit)"=w14) -> ("VISA resource name out"=w10:refnum<visa-resource-name>, "error out"=w9:errorcluster)  [unwired: 4 in, 7 out]
  n183 = call-poly "VISA Configure Serial Port"("VISA resource name"="Top 3 Harvard Syringe Pump Serial Port", "baud rate (9600)"=u32 115200, "stop bits (10: 1 bit)"=w17) -> ("VISA resource name out"=w12:refnum<visa-resource-name>, "error out"=w11:errorcluster)  [unwired: 4 in, 7 out]
  n184 = call-poly "VISA Configure Serial Port"("VISA resource name"="Sample Chamber Stage Serial Port") -> ("VISA resource name out"=w90:refnum<visa-resource-name>, "error out"=w91:errorcluster)  [unwired: 5 in, 8 out]
  "Stage Control Serial Error" <- w91
  n185 = call-poly "VISA Configure Serial Port"("VISA resource name"="Center Harvard Syringe Pump Serial Port", "baud rate (9600)"=u32 115200, "stop bits (10: 1 bit)"=w74) -> ("VISA resource name out"=w71:refnum<visa-resource-name>, "error out"=w72:errorcluster)  [unwired: 4 in, 7 out]
  n186 = node-c288() -> (w101:T22)  [unwired: 4 out]
  n187 = node-c288() -> (w86:T22)  [unwired: 4 in]
  n188 = disable-structure shown="Disabled" {
    disable-tunnel: [w337 _] -> w236
    disable-tunnel: w8 -> [w336 _]
    frame Disabled {
      n189 = node-c288() -> (w339:T22)  [unwired: 4 out]
      n190 = timed-loop "Rough control of MCL mirror stage (debugging)" {
        tunnel: w336 -> [w342]
        tunnel: [w341] -> w337
        timing: w339 -> [_]
        timing-out: [_] -> w338
        stop <- w341 stop-if-true
        n191 = node-c288() -> ()  [unwired: 2 out]
        n192 = case shown="1" "MCL Mode" {
          tunnel: w342 -> [_ w345 w392]
          frame 0, Default {
          }
          frame 1 {
            n193 = node-c288() -> (w347:T22)  [unwired: 4 out]
            n194 = timed-loop "Oscillate MCL mirror" {
              timing: w347 -> [_]
              timing-out: [_] -> w346
              tunnel: w345 -> [w386]
              i -> [w385]
              stop <- w348 stop-if-true
              n195 = node-c288() -> (w384:i64)  [unwired: 1 out]
              n196 = Multiply(x="AO1", y=32767.0) -> (x*y=w380:dbl)
              n197 = Multiply(x="AO2", y=32767.0) -> (x*y=w375:dbl)
              n198 = Divide(x=w380, y=10.0) -> (x/y=w381:dbl)
              n199 = Divide(x=w375, y=10.0) -> (x/y=w376:dbl)
              n200 = To Word Integer(number=w381) -> (16bit integer=w373:i16)
              n201 = To Word Integer(number=w376) -> (16bit integer=w372:i16)
              n202 = Divide(x=w384, y=i64 1000) -> (x/y=w355:dbl)
              n203 = Multiply(x=w355, y=w385) -> (x*y=w366:dbl)
              n204 = Multiply(x="Osc. freq. (Hz) 2", y=6.283185307179586) -> (x*y=w367:dbl)
              n205 = Multiply(x=w367, y=w366) -> (x*y=w365:dbl)
              n206 = Sine(x=w365) -> (sin(x)=w364:dbl)
              n207 = Multiply(x=w364, y="Osc. amp. (V)") -> (x*y=w362:dbl)
              n208 = Add(x=w362, y="Osc. center (V)") -> (x+y=w360:dbl)
              n209 = Divide(x=w360, y=10.0) -> (x/y=w358:dbl)
              n210 = Multiply(x=w358, y=32767.0) -> (x*y=w353:dbl)
              n211 = Select(t=w353, s="Scan axis", f=w373) -> (s? t:f=w371:dbl)
              n212 = Select(t=w372, s="Scan axis", f=w353) -> (s? t:f=w370:dbl)
              n213 = local read "MCL Mode"() -> (w352:u16)
              n214 = Not Equal?(x=w352, y=u16 1) -> (x != y?=w349:bool)
              n215 = local read "Stop All"() -> (w350:bool)
              n216 = xnode "Read/Write Control"("FPGA VI Reference In"=w386, "AO1"=w371, "AO2"=w370) -> ()  [unwired: 1 in, 2 out]
              n217 = Compound Arithmetic op=OR(w350, w349) -> (w348:bool)
              n218 = node-c288() -> ()  [unwired: 2 out]
            }
            n219 = node-c288(w346) -> ()  [unwired: 1 out]
          }
          frame 2 {
            n220 = case shown="True" "Start Scan" {
              tunnel: w392 -> [_ w404]
              frame False {
              }
              frame True {
                n221 = Subtract(x="End (V)", y="Begin (V)") -> (x-y=w400:dbl)
                n222 = Decrement(x="N Points") -> (x-1=w399:dbl)
                n223 = Divide(x=w400, y=w399) -> (x/y=w397:dbl)
                n224 = for {
                  N: "N Points" -> [_]
                  tunnel: "Begin (V)" -> [w417]
                  tunnel: w404 -> [w409]
                  tunnel: [w408] -> w403 mode=indexing
                  tunnel: w397 -> [w407]
                  tunnel: [w405] -> w396 mode=indexing
                  i -> [w416]
                  n225 = Multiply(x=w407, y=w416) -> (x*y=w415:dbl)
                  n226 = Add(x=w417, y=w415) -> (x+y=w412:dbl)
                  n227 = local read "Scan axis"() -> (w406:bool)
                  n228 = local read "AO1"() -> (w414:dbl)
                  n229 = local read "AO2"() -> (w413:dbl)
                  n230 = Select(t=w412, s=w406, f=w414) -> (s? t:f=w411:dbl)
                  n231 = Select(t=w413, s=w406, f=w412) -> (s? t:f=w410:dbl)
                  n232 = flat-sequence {
                    tunnel: w411 -> [w421]
                    tunnel: w410 -> [w420]
                    tunnel: w409 -> [w418]
                    tunnel: [w431] -> w408
                    tunnel: [w430] -> w405
                    frame #0 {
                      w424 = 10.0 ("y")
                      w419 = 32767.0 ("y")
                      n233 = Multiply(x=w421, y=w419) -> (x*y=w427:dbl)
                      n234 = Multiply(x=w420, y=w419) -> (x*y=w425:dbl)
                      n235 = Divide(x=w427, y=w424) -> (x/y=w428:dbl)
                      n236 = Divide(x=w425, y=w424) -> (x/y=w426:dbl)
                      n237 = To Word Integer(number=w428) -> (16bit integer=w422:i16)
                      n238 = To Word Integer(number=w426) -> (16bit integer=w423:i16)
                      n239 = xnode "Read/Write Control"("FPGA VI Reference In"=w418, "AO1"=w422, "AO2"=w423) -> ()  [unwired: 1 in, 2 out]
                    }
                    frame #1 {
                      n240 = Wait (ms)(milliseconds to wait="DAQ Delay (ms)") -> ()  [unwired: 1 out]
                    }
                    frame #2 {
                      n241 = local read "Slow mean"() -> (w431:dbl)
                      n242 = local read "Sigma"() -> (w430:dbl)
                    }
                  }
                }
                n243 = Bundle("Begin (V)"="Begin (V)", w397, w403) -> (→"MCL Scan":cluster{"Begin (V)":dbl, dbl, dbl[]})  [unwired: 1 out]
                n244 = Bundle("Begin (V)"="Begin (V)", w397, w396) -> (→"MCL Scan 2":cluster{"Begin (V)":dbl, dbl, dbl[]})  [unwired: 1 out]
              }
            }
          }
        }
        n245 = local read "Stop All"() -> (w341:bool)
        n246 = node-c288() -> ()  [unwired: 2 out]
      }
      n247 = node-c288(w338) -> ()  [unwired: 1 out]
    }
    frame Enabled {
    }
  }
  n248 = node-c288(i64 1 ("Period"), 1 ("Processor")) -> (w181:T22)  [unwired: 2 out]
  n249 = node-c288(2 ("Processor")) -> (w99:T22)  [unwired: 3 out]
  n250 = timed-loop "Mouse control: trap position (AOM deflection), set confocal spot from image" {
    tunnel: [w435] -> w188
    tunnel: w8 -> [w434]
    timing: w101 -> [_]
    timing-out: [_] -> w100
    stop <- w435 stop-if-true
    n251 = node-c288() -> ()  [unwired: 2 out]
    n252 = event shown="[0] \"Pane\": Mouse Down" {
      selector: _ -> [_ _]
      dyn-events: _ -> [_ _]
      timeout: _ -> [_ _]
      tunnel: w434 -> [w438 _]
      event Mouse Down {
        n253 = event-data() -> ("Time"=w440:u32, "Coords"=w439:T8, "Button"=w441:u16)  [unwired: 6 out]
        n254 = case shown="1" w441 {
          tunnel: w440 -> [_ _ w547]
          tunnel: w439 -> [_ w478 w545]
          tunnel: w438 -> [_ _ w543]
          frame 0, Default {
          }
          frame 1 {
            n255 = property on="APD 2" class="ImageControl"() -> ("Displayed Image Position"=w448:cluster{"Left":i32, "Top":i32})  [unwired: 2 in, 2 out]
            n256 = property on="APD 1" class="ImageControl"() -> ("Displayed Image Position"=w477:cluster{"Left":i32, "Top":i32})  [unwired: 2 in, 2 out]
            n257 = property on="Detection Laser X" class="ImageControl"() -> ("Displayed Image Position"=w474:cluster{"Left":i32, "Top":i32})  [unwired: 2 in, 2 out]
            n258 = property on="Detection Laser Y" class="ImageControl"() -> ("Displayed Image Position"=w473:cluster{"Left":i32, "Top":i32})  [unwired: 2 in, 2 out]
            n259 = property on="APD 2" class="ImageControl"() -> ("Displayed Image Size"=w447:cluster{"Width":u32, "Height":u32})  [unwired: 2 in, 2 out]
            n260 = property on="APD 1" class="ImageControl"() -> ("Displayed Image Size"=w475:cluster{"Width":u32, "Height":u32})  [unwired: 2 in, 2 out]
            n261 = property on="Detection Laser X" class="ImageControl"() -> ("Displayed Image Size"=w476:cluster{"Width":u32, "Height":u32})  [unwired: 2 in, 2 out]
            n262 = property on="Detection Laser Y" class="ImageControl"() -> ("Displayed Image Size"=w472:cluster{"Width":u32, "Height":u32})  [unwired: 2 in, 2 out]
            n263 = Unbundle By Name(w447) -> ("Width"=w444:u32, "Height"=w443:u32)
            n264 = Unbundle By Name(w448) -> ("Left"=w446:i32, "Top"=w445:i32)
            n265 = Unbundle By Name(w475) -> ("Width"=w469:u32, "Height"=w468:u32)
            n266 = Unbundle By Name(w476) -> ("Width"=w465:u32, "Height"=w464:u32)
            n267 = Unbundle By Name(w472) -> ("Width"=w461:u32, "Height"=w460:u32)
            n268 = Unbundle By Name(w477) -> ("Left"=w471:i32, "Top"=w470:i32)
            n269 = Unbundle By Name(w474) -> ("Left"=w467:i32, "Top"=w466:i32)
            n270 = Unbundle By Name(w473) -> ("Left"=w463:i32, "Top"=w462:i32)
            n271 = Bundle("Left"=w446, "Top"=w445, "Width"=w444, "Height"=w443) -> (w442:T25)  [unwired: 1 in]
            n272 = Bundle("Left"=w471, "Top"=w470, "Width"=w469, "Height"=w468) -> (w459:T25)  [unwired: 1 in]
            n273 = Bundle("Left"=w467, "Top"=w466, "Width"=w465, "Height"=w464) -> (w458:T25)  [unwired: 1 in]
            n274 = Bundle("Left"=w463, "Top"=w462, "Width"=w461, "Height"=w460) -> (w457:T25)  [unwired: 1 in]
            n275 = Build Cluster Array(w442, w459, w458, w457) -> (w456:T26)
            n276 = for {
              tunnel: w478 -> [w489]
              tunnel: w456 -> [w490] mode=indexing
              shift-right: [w487] -> w454
              shift-left: TRUE -> [w488]
              shift-right: [w486] -> w452
              shift-left: _ -> [w482]
              shift-right: [w485] -> w451
              shift-left: _ -> [w481]
              shift-right: [w484] -> w450
              shift-left: _ -> [w480]
              shift-right: [w483] -> w449
              shift-left: _ -> [w479]
              n277 = case shown="True" w488 {
                selector: w488 -> [w495 _]
                tunnel: w490 -> [_ w504]
                tunnel: w489 -> [_ w502]
                tunnel: [w495 w500] -> w487
                tunnel: [w494 w499] -> w486
                tunnel: [w493 w498] -> w485
                tunnel: [w492 w497] -> w484
                tunnel: [w491 w496] -> w483
                tunnel: w482 -> [w494 _]
                tunnel: w481 -> [w493 _]
                tunnel: w480 -> [w492 _]
                tunnel: w479 -> [w491 _]
                frame False {
                }
                frame True {
                  n278 = Unbundle(w504) -> (w503:T25)
                  n279 = call "isclickinwindow.vi"("Image Param"=w503, "Point32"=w502) -> ("4 Y"=w496:i32, "3 Height"=w497:i32, "2 X"=w498:i32, "1 Width"=w499:i32, "In image?"=w501:bool)  [unwired: 1 in]
                  n280 = Not(x=w501) -> (.not. x?=w500:bool)
                }
              }
            }
            n281 = Not(x=w454) -> (.not. x?=w453:bool)
            n282 = case shown="True" w453 {
              tunnel: w451 -> [_ w518]
              tunnel: w449 -> [_ w517]
              tunnel: w452 -> [_ w516]
              tunnel: w450 -> [_ w515]
              frame False {
              }
              frame True {
                w505 = FALSE ("Get Point")
